vi "HFRR ADV v05.vi"() -> ()   [LabVIEW 2025] (continued)
                        n2289 = property on="Frictional Force ( N )" class="WFChart (strict)"("History Data"=w3345) -> ()  [unwired: 2 in, 2 out]
                        n2290 = property on="Coefficient of Friction" class="WFChart (strict)"("History Data"=w3345) -> ()  [unwired: 2 in, 2 out]
                        n2291 = property on="Frictional Force ( N )" class="WFChart (strict)"("History Data"=w3345) -> ()  [unwired: 2 in, 2 out]
                        n2292 = property on="Electrical Contact Resistance ( % )" class="WFChart (strict)"("History Data"=w3345) -> ()  [unwired: 2 in, 2 out]
                        n2293 = property on="Humidity ( %RH )" class="WFChart (strict)"("History Data"=w3345) -> ()  [unwired: 2 in, 2 out]
                        n2294 = property on="Stroke ( mm )" class="WFChart (strict)"("History Data"=w3346) -> ()  [unwired: 2 in, 2 out]
                        n2295 = property on="Temperature ( Deg C )" class="WFChart (strict)"("History Data"=w3345) -> ()  [unwired: 2 in, 2 out]
                        n2296 = property on="Service Password Log" class="Str"("Visible"=w3347) -> ()  [unwired: 2 in, 2 out]
                        n2297 = property on="Password 3" class="Clust (strict)"("Visible"=w3347) -> ()  [unwired: 2 in, 2 out]
                      }
                    }
                    "TEST FILE NAM,E SAVED" <- TRUE ("TEST FILE NAM,E SAVED")
                  }
                }
              }
            }
          }
        }
        n2298 = case shown="True" w2659 {
          frame False {
            n2299 = local write "tfalg"(0.0 ("tfalg")) -> ()
          }
          frame True {
            n2300 = local read "tfalg"() -> (w2804:dbl)
            n2301 = Equal?(x=w2804, y=0.0) -> (x = y?=w2805:bool)
            n2302 = case shown="True" w2805 {
              frame False {
              }
              frame True {
                n2303 = local read "Total No. of Tests"() -> (w2808:dbl)
                n2304 = local write "tfalg"(1.0 ("tfalg")) -> ()
                n2305 = local write "acq 2"(FALSE ("acq 2")) -> ()
                n2306 = Wait (ms)(milliseconds to wait=u32 200) -> ()  [unwired: 1 out]
                n2307 = Increment(x=w2808) -> (x+1=w2807:dbl)
                n2308 = local write "Total No. of Tests"(w2807) -> ()
              }
            }
          }
        }
        n2309 = local write "Test \nStatus"(w2665) -> ()
        n2310 = local write "Save"(w2665) -> ()
        n2311 = local read "Main Tab"() -> (w2622:T2)
        n2312 = case shown="True" w2646 {
          tunnel: [FALSE ("RUN") TRUE ("RUN")] -> w2645
          tunnel: [_ 1] -> w2638
          frame False {
          }
          frame True {
          }
        }
        n2313 = In Range and Coerce(upper limit=w2653, x=w2626, lower limit=w2652) -> (In Range?=w2644:bool)  [unwired: 1 out]
        n2314 = In Range and Coerce(upper limit=w2650, x=w2625, lower limit=w2651) -> (In Range?=w2642:bool)  [unwired: 1 out]
        n2315 = case shown="True" w2658 {
          frame False {
            n2316 = local read "Rt 3"() -> (w2786:bool)
            n2317 = case shown="True" w2786 {
              frame False {
              }
              frame True {
                n2318 = local write "Rt 3"(FALSE ("Rt 3")) -> ()
                n2319 = local write "Json End Flg"(TRUE ("Upld AR 2")) -> ()
              }
            }
            "Rt" <- TRUE ("Rt")
            "Rt 2" <- FALSE ("Rt")
          }
          frame True {
            n2320 = local read "Rt"() -> (w2793:bool)
            n2321 = local write "Rt 2"(TRUE ("Rt 2")) -> ()
            n2322 = case shown="True" w2793 {
              frame False {
              }
              frame True {
                w2794 = TRUE ("Upld AR 2")
                n2323 = local write "Rt"(FALSE ("Rt")) -> ()
                n2324 = local write "Upld AR"(w2794) -> ()
                n2325 = local write "Json St Flg"(w2794) -> ()
              }
            }
            "Rt 3" <- TRUE ("Rt 3")
          }
        }
        n2326 = case shown="True" w2644 {
          tunnel: [FALSE ("RUN") TRUE ("RUN")] -> w2643
          tunnel: [_ 2] -> w2637
          frame False {
          }
          frame True {
          }
        }
        n2327 = case shown="True" w2642 {
          tunnel: [FALSE ("RUN") TRUE ("RUN")] -> w2641
          tunnel: [_ 3] -> w2636
          frame False {
          }
          frame True {
          }
        }
        n2328 = case shown="\"Acquire\"" w2622 {
          tunnel: w2624 -> [_ w2855]
          frame Default {
            w2854 = 0.0 ("output")
            n2329 = local write "PID-out"(w2854) -> ()
            n2330 = local write "Frequency ( Hz )"(w2854) -> ()
          }
          frame "Acquire" {
            n2331 = stacked-sequence {
              frame #0 {
                n2332 = local read "Auto Start Test"() -> (w2860:bool)
                n2333 = case shown="True" w2860 {
                  tunnel: "RUN" -> [w2880 w2883]
                  tunnel: [w2880 w2882] -> w2861
                  frame False {
                  }
                  frame True {
                    n2334 = local read "Auto Start Temp"() -> (w2881:bool)
                    n2335 = Or(x=w2883, y=w2881) -> (x .or. y?=w2882:bool)
                  }
                }
                n2336 = local read "clk"() -> (w2879:dbl)
                n2337 = local read "Save"() -> (w2875:bool)
                n2338 = Equal?(x=w2879, y=0.0) -> (x = y?=w2876:bool)
                n2339 = And(x=w2876, y=w2875) -> (x .and. y?=w2877:bool)
                n2340 = Not(x="Engage") -> (.not. x?=w2866:bool)
                n2341 = case shown="True" w2861 {
                  tunnel: [0.0 w2900] -> w2858
                  frame False {
                    (unwired) TRUE ("Visible")
                    n2342 = local read "Auto Start Test"() -> (w2887:bool)
                    n2343 = local write "Start Time"(TRUE ("Start Time")) -> ()
                    n2344 = property on="Stroke 2" class="DigNum (strict)"("Visible"=FALSE) -> ()  [unwired: 2 in, 2 out]
                    n2345 = case shown="False" w2887 {
                      frame False {
                        n2346 = property on="Heater Button" class="Bool (strict)"("DisabledEnum"=T13."Enabled" ("Disabled")) -> ()  [unwired: 2 in, 2 out]
                        n2347 = property on="Humidity" class="Bool (strict)"("DisabledEnum"=T13."Enabled" ("Disabled")) -> ()  [unwired: 2 in, 2 out]
                      }
                      frame True {
                      }
                    }
                    n2348 = case shown="False" "TestCompFlg" {
                      frame False {
                        n2349 = local read "StartFlg"() -> (w2895:bool)
                        n2350 = case shown="True" w2895 {
                          frame False {
                          }
                          frame True {
                            n2351 = flat-sequence {
                              frame #0 {
                                n2352 = local read "EVENT LOG"() -> (w2897:string)
                                n2353 = call "Event Log.vi"("Content"="Test was interrupted", "EVENT LOG"=w2897) -> ("EVENT LOG"=w2898:string)  [unwired: 8 in, 1 out]
                                n2354 = local write "EVENT LOG"(w2898) -> ()
                              }
                              frame #1 {
                                w2899 = FALSE ("StartFlg")
                                n2355 = local write "Heater Button"(w2899) -> ()
                                n2356 = local write "StartFlg"(w2899) -> ()
                                n2357 = local write "Humidity"(w2899) -> ()
                              }
                            }
                          }
                        }
                      }
                      frame True {
                      }
                    }
                    n2358 = local write "String 14"("Test will autostart once parameters reach the set value." ("String 14")) -> ()
                  }
                  frame True {
                    (unwired) FALSE ("Visible")
                    n2359 = property on="Stroke 2" class="DigNum (strict)"("Visible"=TRUE) -> ()  [unwired: 2 in, 2 out]
                    n2360 = property on="STOP 2" class="Bool (strict)"("Disabled"=u8 2) -> ()  [unwired: 2 in, 2 out]
                    n2361 = local write "String 14"(" Running....." ("String 14")) -> ()
                    n2362 = property on="Heater Button" class="Bool (strict)"("DisabledEnum"=T13."Disabled and Grayed Out" ("Disabled")) -> ()  [unwired: 2 in, 2 out]
                    n2363 = property on="Humidity" class="Bool (strict)"("DisabledEnum"=T13."Disabled and Grayed Out" ("Disabled")) -> ()  [unwired: 2 in, 2 out]
                    n2364 = case shown="True" "Start Time" {
                      selector: "Start Time" -> [_ w2913]
                      frame False {
                      }
                      frame True {
                        n2365 = Not(x=w2913) -> (.not. x?=w2912:bool)
                        n2366 = local write "Start Time"(w2912) -> ()
                        n2367 = local read "EVENT LOG"() -> (w2914:string)
                        n2368 = call "Event Log.vi"("Content"="Test in progress", "EVENT LOG"=w2914) -> ("EVENT LOG"=w2916:string)  [unwired: 8 in, 1 out]
                        n2369 = local write "EVENT LOG"(w2916) -> ()
                      }
                    }
                    n2370 = local read "Set Hz"() -> (w2910:dbl)
                    n2371 = call <vilib>:"Uniform White Noise Waveform.vi"() -> ("signal out"=w2909:waveform(dbl))  [unwired: 10 in, 1 out]
                    n2372 = Add(x=w2910, y=w2909) -> (x+y=w2908:waveform(dbl))
                    n2373 = Multiply(x=w2908, y=ext 0.1) -> (x*y=w2900:waveform(ext))
                    "StartFlg" <- TRUE ("StartFlg")
                  }
                }
                n2374 = case shown="True" w2877 {
                  frame False {
                  }
                  frame True {
                    n2375 = local write "clk"(10.0 ("clk")) -> ()
                    n2376 = Get Date/Time In Seconds() -> (seconds since 1Jan1904=w2919:timestamp)
                    n2377 = To Double Precision Float(number=w2919) -> (double precision float=w2917:dbl)
                    n2378 = local write "acq timer"(w2917) -> ()
                    n2379 = local write "act save time"(w2917) -> ()
                  }
                }
                n2380 = call "Elapsed Time"("Time Target (s)"="Countdown", "Reset"=w2866) -> ("Elapsed Time (s)"=w2871:dbl, "Time has Elapsed"=w2869:bool)  [unwired: 10 in, 6 out]
                "Countdown 2" <- w2871
                n2381 = Subtract(x=w2871, y=2.0) -> (x-y=w2874:dbl)
                n2382 = Less?(x=w2874, y="Countdown") -> (x < y?=w2872:bool)
                n2383 = And(x=w2872, y=w2869) -> (x .and. y?=w2868:bool)
                n2384 = case shown="True" w2868 {
                  frame False {
                  }
                  frame True {
                    (unwired) dbl[] [] ("History Data")
                    n2385 = local write "Engage"(FALSE ("Engage")) -> ()
                    n2386 = local write "RUN"(TRUE ("RUN")) -> ()
                    n2387 = local read "Humidity ( %RH )"() -> (→"Rh Before":dbl)
                  }
                }
                n2388 = local read "Test \nStatus"() -> (w2864:bool)
                n2389 = Multiply(x=w2858, y=10.0) -> (x*y=w2859:dbl)
                n2390 = Select(t=w2859, s=w2864, f=0.0) -> (s? t:f=w2863:dbl)
                n2391 = local write "Frequency ( Hz )"(w2863) -> ()
              }
              frame #1 {
                w2942 = 1000000.0 ("x")
                # "Elapsed time\ncof\nstroke\nAir temp\nTemp\nHumidity"
                # "acq timer\n\nact save time"
                # "convert to microseconds"
                n2392 = local read "COUNT"() -> (w2925:i32)
                n2393 = local read "Rate"() -> (w2938:dbl)
                n2394 = Divide(x=w2942, y=w2938) -> (x/y=w2943:dbl)
                n2395 = Greater Or Equal?(x=w2925, y=250) -> (x >= y?=w2924:bool)
                n2396 = Get Date/Time In Seconds() -> (seconds since 1Jan1904=w2945:timestamp)
                n2397 = case shown="True" w2924 {
                  frame False {
                    n2398 = local read "COUNT"() -> (w2946:i32)
                    n2399 = Increment(x=w2946) -> (x+1=w2947:i32)
                    n2400 = local write "COUNT"(w2947) -> ()
                  }
                  frame True {
                    n2401 = local write "COUNT"(0 ("COUNT")) -> ()
                  }
                }
                n2402 = local read "Samplingtime 2"() -> (w2923:dbl)
                n2403 = local read "act save time"() -> (w2940:dbl)
                n2404 = Divide(x=w2943, y=w2942) -> (x/y=w2941:dbl)
                n2405 = To Double Precision Float(number=w2945) -> (double precision float=w2934:dbl)
                n2406 = Add(x=w2940, y=w2923) -> (x+y=w2939:dbl)
                n2407 = local read "acq timer"() -> (w2944:dbl)
                n2408 = local read "COUNT"() -> (w2927:i32)
                n2409 = Greater Or Equal?(x=w2934, y=w2939) -> (x >= y?=w2922:bool)
                n2410 = Multiply(x=w2941, y=w2927) -> (x*y=w2933:dbl)
                n2411 = Subtract(x=w2934, y=w2944) -> (x-y=w2936:dbl)
                n2412 = local read "Save"() -> (w2937:bool)
                n2413 = Add(x=w2936, y=w2933) -> (x+y=w2920:dbl)
                "Elapsed time 3" <- w2920
                n2414 = And(x=w2922, y=w2937) -> (x .and. y?=w2935:bool)
                n2415 = Divide(x=w2920, y=60.0) -> (x/y=w2931:dbl)
                n2416 = local read "Test \nStatus"() -> (w2921:bool)
                n2417 = local read "clk"() -> (w2928:dbl)
                n2418 = Equal?(x=w2928, y=10.0) -> (x = y?=w2930:bool)
                n2419 = case shown="True" w2935 {
                  tunnel: w2934 -> [_ w3051]
                  tunnel: [FALSE ("Boolean 2") TRUE ("Boolean 2")] -> _
                  frame False {
                  }
                  frame True {
                    w3005 = ";" ("Substring")
                    # "Pid out/\nFreq response value"
                    n2420 = local write "act save time"(w3051) -> ()
                    n2421 = local read "FILE"() -> (w2999:string)
                    n2422 = call "file check.vi"("file name in"=w2999) -> ("error out"=w3002:errorcluster, "file name out"=w2997:string)  [unwired: 9 in]
                    n2423 = call "FILE PATH CREATION.vi"("error in"=w3002, "FILE NAME :"=w2997) -> ("FILE OUT"=w3000:path)  [unwired: 8 in, 1 out]
                    n2424 = Concatenate Strings(w2997, ".dgf" ("Substring")) -> (w3001:string)
                    n2425 = local read "FF 2"() -> (→"Frictional Force ( N )" →"Frictional Force ( N )":dbl)
                    n2426 = Build Path(base path=w3000, name or relative path=w3001) -> (appended path=w2996:path)
                    n2427 = local read "COF 2"() -> (w3010:dbl)
                    "cof" <- w3010
                    "Coefficient of Friction" <- w3010
                    "COF 4" <- w3010
                    "Coefficient of Friction" <- w3010
                    n2428 = local read "TEMP"() -> (w3013:dbl)
                    "Temp" <- w3013
                    "Temperature ( Deg C )" <- w3013
                    n2429 = local read "Humidity ( %RH )"() -> (w3012:dbl)
                    "Humidity ( %RH )" <- w3012
                    "Humidity ( %RH )" <- w3012
                    n2430 = local read "Frequency ( Hz )"() -> (w3019:dbl)
                    n2431 = local read "Elapsed time"() -> (w3044:dbl)
                    n2432 = local read "AIR TEMP"() -> (w3017:dbl)
                    n2433 = local read "PID-out"() -> (w3022:dbl)
                    n2434 = local write "Temperature ( Deg C )"(w3013) -> ()
                    n2435 = Number To Fractional String(number="measured_stroke", width (-)=i16 9 ("precision (6)"), precision (6)=i16 6) -> (F-format string=w3037:string)  [unwired: 1 in]
                    n2436 = Number To Fractional String(number=w3017, width (-)=i16 9 ("precision (6)"), precision (6)=i16 3) -> (F-format string=w3036:string)  [unwired: 1 in]
                    n2437 = Number To Fractional String(number=w3013, width (-)=i16 9 ("precision (6)"), precision (6)=i16 3) -> (F-format string=w3033:string)  [unwired: 1 in]
                    n2438 = Number To Fractional String(number=w3012, width (-)=i16 9 ("precision (6)"), precision (6)=i16 3) -> (F-format string=w3030:string)  [unwired: 1 in]
                    n2439 = Number To Fractional String(number=0.0, width (-)=i16 9 ("precision (6)"), precision (6)=i16 3) -> (F-format string=w3027:string)  [unwired: 1 in]
                    n2440 = Number To Fractional String(number=w3022, width (-)=i16 9 ("precision (6)"), precision (6)=i16 3) -> (F-format string=w3023:string)  [unwired: 1 in]
                    n2441 = Number To Fractional String(number=w3019, width (-)=i16 9 ("precision (6)"), precision (6)=i16 3) -> (F-format string=w3018:string)  [unwired: 1 in]
                    n2442 = Number To Fractional String(number=w3010, width (-)=i16 9 ("precision (6)"), precision (6)=i16 6) -> (F-format string=w3045:string)  [unwired: 1 in]
                    n2443 = Number To Fractional String(number=w3044, width (-)=i16 14 ("precision (6)"), precision (6)=i16 3) -> (F-format string=w3046:string)  [unwired: 1 in]
                    n2444 = Bundle("y"=1.02, "measured_stroke"="measured_stroke", "y"=0.98) -> (w3011:cluster{"y":dbl, "measured_stroke":dbl, "y":dbl})  [unwired: 1 in]
                    n2445 = Number To Fractional String(number="Ambient Humidity :", width (-)=i16 9 ("precision (6)"), precision (6)=i16 6) -> (F-format string=w3003:string)  [unwired: 1 in]
                    n2446 = local read "RUN"() -> (w3009:bool)
                    n2447 = case shown="True" w3009 {
                      tunnel: w3011 -> [_ w3056]
                      tunnel: "measured_stroke" -> [_ w3055]
                      tunnel: "measured_stroke" -> [_ w3054]
                      tunnel: "measured_stroke" -> [_ w3053]
                      frame False {
                      }
                      frame True {
                        "Stroke ( mm )" <- w3056
                        "Stroke ( mm )" <- w3056
                        "Stroke 4" <- w3055
                        "Stroke 3" <- w3054
                        "Stroke 2" <- w3053
                      }
                    }
                    n2448 = Concatenate Strings(w3046, w3005, w3045, w3005, w3037, w3005, w3036, w3005, w3033, w3005, w3030, w3005, w3027, w3005, w3023, w3005, w3018, w3005, w3003, "\r") -> (w3043:string)
                    n2449 = call <vilib>:"Write Characters To File.vi"("append to file? (new file:F)"=TRUE, "character string"=w3043, "file path (dialog if empty)"=w2996) -> ()  [unwired: 2 in, 1 out]
                    "refresh flag" <- TRUE ("refresh flag")
                  }
                }
                n2450 = case shown="True" w2921 {
                  tunnel: w2931 -> [_ w2957]
                  tunnel: w2936 -> [_ w2967]
                  tunnel: [0.0 w2963] -> _
                  tunnel: w2930 -> [_ w2962]
                  tunnel: [0.0 w2961] -> _
                  tunnel: w2920 -> [_ w2961]
                  tunnel: w2934 -> [w2950 _]
                  frame False {
                    n2451 = local write "acq timer"(w2950) -> ()
                    n2452 = local write "Test Duration Status"(0.0 ("Test Duration Status")) -> ()
                  }
                  frame True {
                    n2453 = local read "Set Hz"() -> (w2964:dbl)
                    n2454 = local write "Elapsed time"(w2957) -> ()
                    n2455 = local read "test time"() -> (w2956:dbl)
                    n2456 = Multiply(x=w2967, y=w2964) -> (x*y=w2966:dbl)
                    n2457 = case shown="False" w2962 {
                      tunnel: w2966 -> [w2968 _]
                      tunnel: [w2968 1.0] -> w2963
                      frame False {
                        n2458 = local write "Cycles elapsed"(w2968) -> ()
                      }
                      frame True {
                      }
                    }
                    n2459 = Greater?(x=w2957, y=w2956) -> (0:w2965:bool)
                    n2460 = Subtract(x=w2956, y=w2957) -> (x-y=w2955:dbl)
                    "time" <- w2955
                    n2461 = Multiply(x=w2955, y=60.0) -> (x*y=w2954:dbl)
                    n2462 = local write "Time Remaining"(w2954) -> ()
                    n2463 = local write "Remaining Time"(w2954) -> ()
                    n2464 = case shown="True" w2965 {
                      frame False {
                      }
                      frame True {
                        n2465 = stacked-sequence {
                          frame #0 {
                            w2971 = T13."Enabled" ("Disabled")
                            w2970 = FALSE ("TEST FILE NAM,E SAVED")
                            w2974 = "" ("FILE")
                            w2975 = TRUE ("Visible")
                            n2466 = local write "Humidity"(FALSE ("Humidity")) -> ()
                            n2467 = local write "RUN"(FALSE ("OK Button 2")) -> ()
                            n2468 = local write "Heater Button"(FALSE ("Heater Button")) -> ()
                            n2469 = local write "Auto Start Test"(FALSE ("Auto Start Test")) -> ()
                            n2470 = local write "TestCompFlg"(TRUE ("StpFlg")) -> ()
                            n2471 = local read "Humidity ( %RH )"() -> (→"Rh After":dbl)
                            n2472 = property on="STOP 2" class="Bool (strict)"("Disabled"=u8 0) -> ()  [unwired: 2 in, 2 out]
                            n2473 = local read "EVENT LOG"() -> (w2980:string)
                            n2474 = call "Event Log.vi"("Content"="Test Completed", "EVENT LOG"=w2980) -> ("EVENT LOG"=w2979:string)  [unwired: 8 in, 1 out]
                            n2475 = property on="RUN" class="Bool (strict)"("Visible"=w2975) -> ()  [unwired: 2 in, 2 out]
                            n2476 = property on="Auto Start Test" class="Bool (strict)"("Visible"=w2975) -> ()  [unwired: 2 in, 2 out]
                            n2477 = local write "Batch Ref Num :"(w2974) -> ()
                            n2478 = local write "FILE"(w2974) -> ()
                            n2479 = local write "EVENT LOG"(w2979) -> ()
                            n2480 = local write "TEST FILE NAM,E SAVED"(w2970) -> ()
                            n2481 = local write "Fuel Discription :"(w2974) -> ()
                            n2482 = local write "START TEMP"(w2970) -> ()
                            n2483 = local write "Remarks :"(w2974) -> ()
                            n2484 = local write "Main Dashboard Buttons"(T1."Imaging" ("Main Dashboard Buttons")) -> ()
                            n2485 = local write "Main Tab"(T2."Adv Scar" ("Main Tab")) -> ()
                            n2486 = property on="FRICVALZ 2" class="Bool (strict)"("DisabledEnum"=w2971) -> ()  [unwired: 2 in, 2 out]
                            n2487 = property on="FRICVALZ 3" class="Bool (strict)"("DisabledEnum"=w2971) -> ()  [unwired: 2 in, 2 out]
                            n2488 = property on="FRICVALZ 4" class="Bool (strict)"("DisabledEnum"=w2971) -> ()  [unwired: 2 in, 2 out]
                          }
                          frame #1 {
                            n2489 = Wait (ms)(milliseconds to wait=u32 1500) -> ()  [unwired: 1 out]
                          }
                          frame #2 {
                            n2490 = local write "Command"("VC;0") -> ()
                          }
                          frame #3 {
                            n2491 = Wait (ms)(milliseconds to wait=u32 1500) -> ()  [unwired: 1 out]
                          }
                          frame #4 {
                            n2492 = local write "Command"("ST;0") -> ()
                          }
                          frame #5 {
                            n2493 = Wait (ms)(milliseconds to wait=u32 1500) -> ()  [unwired: 1 out]
                          }
                          frame #6 {
                            n2494 = local write "Command"("HE;0" ("Command")) -> ()
                          }
                          frame #7 {
                            n2495 = Wait (ms)(milliseconds to wait=u32 1500) -> ()  [unwired: 1 out]
                          }
                        }
                      }
                    }
                    n2496 = Divide(x=w2957, y=w2956) -> (x/y=w2960:dbl)
                    n2497 = Multiply(x=w2960, y=100.0) -> (x*y=w2958:dbl)
                    n2498 = local write "Test Duration Status"(w2958) -> ()
                  }
                }
              }
              frame #2 {
                n2499 = case shown="True" "Heater Button" {
                  tunnel: [0.0 ("output") w3066] -> w3057
                  frame False {
                    w3060 = TRUE ("tmpchk")
                    n2500 = local read "TEMP"() -> (w3061:dbl)
                    n2501 = local write "Temp ini"(w3061) -> ()
                    n2502 = local write "Reset 4"(w3060) -> ()
                    n2503 = local write "tmpchk"(w3060) -> ()
                    n2504 = local write "reinit"(TRUE ("reinit")) -> ()
                    n2505 = local write "manual temp log"(TRUE ("manual temp log")) -> ()
                  }
                  frame True {
                    n2506 = local read "Auto Start Test"() -> (w3065:bool)
                    n2507 = case shown="True" FALSE {
                      tunnel: [_ w3081] -> w3066
                      frame False {
                      }
                      frame True {
                        # "Logic to turn off\nthe heater when \ntemp is not rising.\nTime - 60 sec\nDelta t- 5°c"
                        n2508 = local read "Temp ini"() -> (w3070:dbl)
                        n2509 = Less?(x=w3070, y=53.0) -> (x < y?=w3068:bool)
                        n2510 = And(x="tmpchk", y=w3068) -> (x .and. y?=w3071:bool)
                        n2511 = case shown="True" w3071 {
                          frame False {
                          }
                          frame True {
                            n2512 = call "Elapsed Time8"("Time Target (s)"=300.0, "Reset"="Reset 4") -> ("Time has Elapsed"=w3084:bool)  [unwired: 10 in, 7 out]
                            n2513 = flat-sequence {
                              tunnel: w3084 -> [_]
                              frame #0 {
                                n2514 = local write "Reset 4"(FALSE ("Reset 4")) -> ()
                              }
                            }
                            n2515 = case shown="True" w3084 {
                              frame False {
                              }
                              frame True {
                                n2516 = local read "Temp ini"() -> (w3091:dbl)
                                n2517 = Add(x=w3091, y=5.0) -> (x+y=w3089:dbl)
                                n2518 = local read "TEMP"() -> (w3092:dbl)
                                n2519 = Greater?(x=w3092, y=w3089) -> (0:w3090:bool)
                                n2520 = case shown="False" w3090 {
                                frame False {
                                n2521 = local write "Heater Button"(FALSE ("Heater Button")) -> ()
                                }
                                frame True {
                                n2522 = local write "tmpchk"(FALSE ("tmpchk")) -> ()
                                }
                                }
                              }
                            }
                          }
                        }
                        n2523 = local read "Set Temp"() -> (w3079:dbl)
                        n2524 = local read "TEMP"() -> (w3073:dbl)
                        n2525 = call-poly <vilib>:"PID.vi"("reinitialize? (F)"="reinit", "dt (s)"=-1.0, "process variable"=w3073, "setpoint"=w3079) -> ("output"=w3076:dbl)  [unwired: 6 in, 1 out]
                        n2526 = Subtract(x=w3079, y=w3073) -> (x-y=w3080:dbl)
                        n2527 = Add(x=w3079, y=0.5) -> (x+y=w3077:dbl)
                        n2528 = Greater Or Equal?(x=w3073, y=w3077) -> ()  [unwired: 1 out]
                        n2529 = Select(t=0.0, s=FALSE, f=w3076) -> (s? t:f=w3075:dbl)
                        "PID output" <- w3075
                        n2530 = flat-sequence {
                          tunnel: w3075 -> [w3095]
                          tunnel: [w3095] -> w3081
                          frame #0 {
                            n2531 = local write "reinit"(FALSE ("reinit")) -> ()
                          }
                        }
                        n2532 = Bundle(w3080, "output"=w3075, "TEMP"=w3073) -> ()  [unwired: 1 in, 1 out]
                      }
                    }
                    n2533 = case shown="False" w3065 {
                      frame False {
                        n2534 = local read "Set Temp"() -> (w3103:dbl)
                        n2535 = local read "TEMP"() -> (w3102:dbl)
                        n2536 = Subtract(x=w3103, y=w3102) -> (x-y=w3101:dbl)
                        n2537 = Absolute Value(x=w3101) -> (abs(x)=w3100:dbl)
                        n2538 = Less?(x=w3100, y=0.5) -> (x < y?=w3098:bool)
                        n2539 = case shown="True" w3098 {
                          tunnel: "manual temp log" -> [_ w3104]
                          frame False {
                          }
                          frame True {
                            n2540 = case shown="True" w3104 {
                              selector: w3104 -> [_ w3105]
                              frame False {
                              }
                              frame True {
                                # "#Event log"
                                n2541 = Not(x=w3105) -> (.not. x?=w3106:bool)
                                n2542 = local write "manual temp log"(w3106) -> ()
                                n2543 = local read "EVENT LOG"() -> (w3109:string)
                                n2544 = call "Event Log.vi"("Content"="Target Temperature reached", "EVENT LOG"=w3109) -> ("EVENT LOG"=w3108:string)  [unwired: 8 in, 1 out]
                                n2545 = local write "EVENT LOG"(w3108) -> ()
                              }
                            }
                          }
                        }
                      }
                      frame True {
                        n2546 = local write "manual temp log"(TRUE ("manual temp log")) -> ()
                      }
                    }
                  }
                }
                "PID-out" <- w3057
              }
              frame #3 {
                n2547 = local read "TEMP"() -> (w3111:dbl)
                n2548 = Greater Or Equal?(x=w3111, y="Set Temp 2") -> (x >= y?=w3116:bool)
                n2549 = case shown="True" w3116 {
                  tunnel: [FALSE TRUE] -> w3114
                  frame False {
                  }
                  frame True {
                  }
                }
                "Status 13" <- w3114
                n2550 = And(x=w3114, y="trip1 8") -> (x .and. y?=w3113:bool)
                n2551 = case shown="True" w3113 {
                  frame False {
                    n2552 = local write "Heater Trip Temp"(TRUE ("Heater Trip Temp")) -> ()
                  }
                  frame True {
                    w3119 = FALSE ("OK Button 2")
                    n2553 = case shown="True" "Heater Trip Temp" {
                      selector: "Heater Trip Temp" -> [_ w3121]
                      frame False {
                      }
                      frame True {
                        n2554 = Not(x=w3121) -> (.not. x?=w3120:bool)
                        n2555 = local read "EVENT LOG"() -> (w3124:string)
                        n2556 = local write "Heater Trip Temp"(w3120) -> ()
                        n2557 = call "Event Log.vi"("Content"="Heater Trip", "EVENT LOG"=w3124) -> ("EVENT LOG"=w3123:string)  [unwired: 8 in, 1 out]
                        n2558 = local write "EVENT LOG"(w3123) -> ()
                      }
                    }
                    n2559 = local write "RUN"(w3119) -> ()
                    n2560 = property on="Auto Start Test" class="Bool (strict)"("Value"=w3119) -> ()  [unwired: 2 in, 2 out]
                    n2561 = local write "Heater Button"(w3119) -> ()
                  }
                }
              }
            }
            n2562 = case shown="False" w2855 {
              frame False {
                n2563 = disable-structure shown="Enabled" {
                  frame Disabled {
                    n2564 = stacked-sequence {
                      frame #0 {
                        n2565 = local write "RUN"(FALSE ("OK Button 2")) -> ()
                      }
                      frame #1 {
                      }
                    }
                  }
                  frame Enabled {
                  }
                }
              }
              frame True {
              }
            }
          }
        }
        n2566 = local read "airtempflg"() -> (w2647:bool)
        n2567 = Or(x=w2647, y=w2645) -> (x .or. y?=w2648:bool)
        n2568 = Insert Into Array(array=string[] ["Air Temperature has reached set value,", "Humidity has reached set value,", "Sample Temperaturehas reached set value,", ""], index=0, new element="") -> (w2633:string[])
        n2569 = Build Array(w2638, w2637, w2636) -> (w2634:i32[])
        n2570 = disable-structure shown="Disabled" {
          disable-tunnel: w2648 -> [w2725 _]
          disable-tunnel: w2643 -> [w2724 _]
          disable-tunnel: w2641 -> [w2723 _]
          frame Disabled {
            n2571 = Compound Arithmetic op=AND(w2725, w2724, w2723) -> ()  [unwired: 1 out]
            n2572 = case shown="True" {
              selector: _ -> [_ _]
              frame False {
              }
              frame True {
                w2726 = FALSE ("autostrtflg")
                n2573 = local write "RUN"(TRUE ("RUN")) -> ()
                n2574 = local write "autostrtflg"(w2726) -> ()
                n2575 = local write "autostart"(w2726) -> ()
                n2576 = local write "String 14"(" Running....." ("String 14")) -> ()
              }
            }
          }
          frame Enabled {
          }
        }
        n2577 = for {
          tunnel: w2634 -> [w2776] mode=indexing
          tunnel: w2633 -> [w2775]
          shift-right: [w2772] -> w2632
          shift-left: "" -> [w2774]
          n2578 = Index Array(array=w2775, index=w2776) -> (element=w2773:string)
          n2579 = Concatenate Strings(w2773, w2774) -> (w2772:string)
        }
        n2580 = local write "autostart 2"(w2632) -> ()
        n2581 = local read "Reset Graph"() -> (w2621:bool)
        n2582 = case shown="True" w2621 {
          selector: w2621 -> [_ w2675]
          frame False {
          }
          frame True {
            w2689 = 0.0 ("X Scale.Range:Maximum")
            n2583 = Not(x=w2675) -> (.not. x?=w2674:bool)
            n2584 = local write "Reset Graph"(w2674) -> ()
            n2585 = property on="Electrical Contact Resistance ( % )" class="WFChart (strict)"("XScale.Maximum"=600.0 ("X Scale.Range:Maximum"), "XScale.Minimum"=0.0 ("X Scale.Range:Minimum"), "YScale.Maximum"=100.0 ("Y Scale.Range:Maximum"), "YScale.Minimum"=0.0 ("Y Scale.Range:Minimum")) -> ()  [unwired: 2 in, 2 out]
            n2586 = property on="Frictional Force ( N )" class="WFChart (strict)"("XScale.Maximum"=600.0 ("X Scale.Range:Maximum"), "XScale.Minimum"=0.0 ("X Scale.Range:Minimum"), "YScale.Maximum"=100.0 ("Y Scale.Range:Maximum"), "YScale.Minimum"=0.0 ("Y Scale.Range:Minimum")) -> ()  [unwired: 2 in, 2 out]
            n2587 = property on="Temperature ( Deg C )" class="WFChart (strict)"("XScale.Maximum"=600.0 ("X Scale.Range:Maximum"), "XScale.Minimum"=0.0 ("X Scale.Range:Minimum"), "YScale.Maximum"=100.0 ("Y Scale.Range:Maximum"), "YScale.Minimum"=0.0 ("Y Scale.Range:Minimum")) -> ()  [unwired: 2 in, 2 out]
            n2588 = property on="Humidity ( %RH )" class="WFChart (strict)"("XScale.Maximum"=600.0 ("X Scale.Range:Maximum"), "XScale.Minimum"=0.0 ("X Scale.Range:Minimum"), "YScale.Maximum"=100.0 ("Y Scale.Range:Maximum"), "YScale.Minimum"=0.0 ("Y Scale.Range:Minimum")) -> ()  [unwired: 2 in, 2 out]
            n2589 = property on="Stroke ( mm )" class="WFChart (strict)"("XScale.Maximum"=600.0 ("X Scale.Range:Maximum"), "XScale.Minimum"=0.0 ("X Scale.Range:Minimum"), "YScale.Maximum"=100.0 ("Y Scale.Range:Maximum"), "YScale.Minimum"=0.0 ("Y Scale.Range:Minimum")) -> ()  [unwired: 2 in, 2 out]
            n2590 = property on="Coefficient of Friction" class="WFChart (strict)"("XScale.Maximum"=600.0 ("X Scale.Range:Maximum"), "XScale.Minimum"=0.0 ("X Scale.Range:Minimum"), "YScale.Maximum"=100.0 ("Y Scale.Range:Maximum"), "YScale.Minimum"=0.0 ("Y Scale.Range:Minimum")) -> ()  [unwired: 2 in, 2 out]
            n2591 = property on="Electrical Contact Resistance ( % )" class="WFChart (strict)"("XScale.Minimum"=0.0 ("X Scale.Range:Minimum"), "XScale.Maximum"=600.0 ("X Scale.Range:Maximum"), "YScale.Minimum"=0.0 ("Y Scale.Range:Minimum"), "YScale.Maximum"=100.0 ("Y Scale.Range:Maximum")) -> ()  [unwired: 2 in, 2 out]
            n2592 = property on="Temperature ( Deg C )" class="WFChart (strict)"("XScale.Minimum"=0.0 ("X Scale.Range:Minimum"), "XScale.Maximum"=600.0 ("X Scale.Range:Maximum"), "YScale.Minimum"=0.0 ("Y Scale.Range:Minimum"), "YScale.Maximum"=100.0 ("Y Scale.Range:Maximum")) -> ()  [unwired: 2 in, 2 out]
            n2593 = property on="Coefficient of Friction" class="WFChart (strict)"("XScale.Minimum"=0.0 ("X Scale.Range:Minimum"), "XScale.Maximum"=600.0 ("X Scale.Range:Maximum"), "YScale.Maximum"=1.0 ("X Scale.Range:Minimum"), "YScale.Minimum"=0.0 ("X Scale.Range:Minimum")) -> ()  [unwired: 2 in, 2 out]
            n2594 = property on="Frictional Force ( N )" class="WFChart (strict)"("XScale.Maximum"=600.0 ("X Scale.Range:Maximum"), "XScale.Minimum"=w2689, "YScale.Maximum"=10.0 ("Y Scale.Range:Maximum"), "YScale.Minimum"=w2689) -> ()  [unwired: 2 in, 2 out]
            n2595 = property on="Stroke ( mm )" class="WFChart (strict)"("XScale.Maximum"=600.0 ("X Scale.Range:Maximum"), "XScale.Minimum"=0.0 ("X Scale.Range:Minimum"), "YScale.Maximum"=100.0 ("Y Scale.Range:Maximum"), "YScale.Minimum"=0.0 ("Y Scale.Range:Minimum")) -> ()  [unwired: 2 in, 2 out]
            n2596 = property on="Humidity ( %RH )" class="WFChart (strict)"("XScale.Maximum"=600.0 ("X Scale.Range:Maximum"), "XScale.Minimum"=0.0 ("X Scale.Range:Minimum"), "YScale.Maximum"=100.0 ("Y Scale.Range:Maximum"), "YScale.Minimum"=0.0 ("Y Scale.Range:Minimum")) -> ()  [unwired: 2 in, 2 out]
          }
        }
      }
      frame "Compare Files" {
        # "Elapsed time\ncof\nstroke\nAir temp\nTemp\nHumidity"
        n2597 = case shown="True" "RSTV1 2" {
          frame False {
          }
          frame True {
            n2598 = property on="Humidity ( %RH )" class="XYGraph (strict)"("Y Scale.Display Format:Precision"=u8 0 ("Y Scale.Format & Precision:Precision")) -> ()  [unwired: 2 in, 2 out]
            n2599 = property on="Humidity ( %RH )" class="XYGraph (strict)"("X Scale.Range:Minimum"=0.0, "X Scale.Range:Maximum"=75.0, "Y Scale.Range:Minimum"=48.0, "Y Scale.Range:Maximum"=58.0) -> ()  [unwired: 2 in, 2 out]
          }
        }
        n2600 = case shown="True" "RST CP 2" {
          frame False {
          }
          frame True {
            n2601 = property on="XY Graph 13" class="XYGraph (strict)"("Y Scale.Display Format:Precision"=u8 0 ("Y Scale.Format & Precision:Precision")) -> ()  [unwired: 2 in, 2 out]
            n2602 = property on="XY Graph 13" class="XYGraph (strict)"("X Scale.Range:Minimum"=0.0, "X Scale.Range:Maximum"=75.0, "Y Scale.Range:Minimum"=0.0, "Y Scale.Range:Maximum"=100.0) -> ()  [unwired: 2 in, 2 out]
          }
        }
        n2603 = case shown="True" "RST CP" {
          frame False {
          }
          frame True {
            n2604 = property on="Sample Temperature ( °C )" class="XYGraph (strict)"("Y Scale.Display Format:Precision"=u8 2 ("Y Scale.Format & Precision:Precision")) -> ()  [unwired: 2 in, 2 out]
            n2605 = property on="Sample Temperature ( °C )" class="XYGraph (strict)"("X Scale.Range:Minimum"=0.0, "X Scale.Range:Maximum"=75.0, "Y Scale.Range:Minimum"=58.0, "Y Scale.Range:Maximum"=62.0) -> ()  [unwired: 2 in, 2 out]
          }
        }
        n2606 = case shown="True" "RSTV1 3" {
          frame False {
          }
          frame True {
            n2607 = property on="Air Temperature  ( °C )" class="XYGraph (strict)"("Y Scale.Display Format:Precision"=u8 2 ("Y Scale.Format & Precision:Precision")) -> ()  [unwired: 2 in, 2 out]
            n2608 = property on="Air Temperature  ( °C )" class="XYGraph (strict)"("X Scale.Range:Minimum"=0.0 ("Y Scale.Range:Minimum"), "X Scale.Range:Maximum"=75.0 ("Y Scale.Range:Maximum"), "Y Scale.Range:Minimum"=20.0 ("X Scale.Range:Minimum"), "Y Scale.Range:Maximum"=26.0 ("X Scale.Range:Maximum")) -> ()  [unwired: 2 in, 2 out]
          }
        }
        n2609 = case shown="True" "RSTV1 4" {
          frame False {
          }
          frame True {
            n2610 = property on="Stroke ( mm )" class="XYGraph (strict)"("Y Scale.Display Format:Precision"=u8 2 ("Y Scale.Format & Precision:Precision")) -> ()  [unwired: 2 in, 2 out]
            n2611 = property on="Stroke ( mm )" class="XYGraph (strict)"("X Scale.Range:Minimum"=0.0 ("Y Scale.Range:Maximum"), "X Scale.Range:Maximum"=75.0 ("X Scale.Range:Minimum"), "Y Scale.Range:Minimum"=0.98, "Y Scale.Range:Maximum"=1.02) -> ()  [unwired: 2 in, 2 out]
          }
        }
        n2612 = case shown="True" "rstv2" {
          frame False {
          }
          frame True {
            n2613 = property on="Coefficient Of Friction" class="XYGraph (strict)"("Y Scale.Display Format:Precision"=u8 3 ("Y Scale.Format & Precision:Precision")) -> ()  [unwired: 2 in, 2 out]
            n2614 = property on="Coefficient Of Friction" class="XYGraph (strict)"("X Scale.Range:Minimum"=0.0 ("Y Scale.Range:Maximum"), "X Scale.Range:Maximum"=75.0, "Y Scale.Range:Minimum"=0.0, "Y Scale.Range:Maximum"=1.0 ("X Scale.Range:Minimum")) -> ()  [unwired: 2 in, 2 out]
          }
        }
        n2615 = case shown="True" "RST CP 3" {
          frame False {
          }
          frame True {
            n2616 = property on="Air Temp ( °C ) vs Humidity ( % RH )" class="XYGraph (strict)"("X Scale.Range:Minimum"=18.0, "X Scale.Range:Maximum"=28.0 ("X Scale.Range:Minimum"), "Y Scale.Range:Minimum"=30.0 ("X Scale.Range:Minimum"), "Y Scale.Range:Maximum"=70.0 ("X Scale.Range:Minimum")) -> ()  [unwired: 2 in, 2 out]
          }
        }
        n2617 = case shown="True" "OPEN 1" {
          frame False {
          }
          frame True {
            (unwired) 0  # existing file
            w3400 = "Choose a datalog file to open"  # prompt
            n2618 = local write "OPEN 1"(FALSE ("OPEN 1")) -> ()
            n2619 = String To Path(string="C:\\LAB-IQ\\Data\\") -> (path=w3385:path)
            n2620 = File Dialog(6:"*.dgf" ("pattern"), 7:w3400, 11:w3385) -> (0:w3383:errorcluster, 3:w3391:path)  [unwired: 4 in, 2 out]
            n2621 = Unbundle(w3383) -> ()  [unwired: 3 out]
            n2622 = Strip Path(path=w3391) -> (name=w3390:string)  [unwired: 1 out]
            n2623 = Path To String(path=w3391) -> (string=w3386:string)
            "string1" <- w3386
            n2624 = Match Pattern(string=w3390, regular expression=".dgf") -> (before substring=→"String Control":string)  [unwired: 1 in, 3 out]
            n2625 = Match Pattern(string=w3386, regular expression=".dgf" ("substring (\"\")")) -> (before substring=w3396:string)  [unwired: 1 in, 3 out]
            n2626 = Concatenate Strings(w3396, ".duf" ("Substring")) -> (w3392:string)
            n2627 = String To Path(string=w3392) -> (path=w3397:path)
            n2628 = call <vilib>:"Read Characters From File.vi"("file path (dialog if empty)"=w3397, "start of read offset (chars.:0)"=60 ("start of read offset (chars.: 0)")) -> ("character string"=→"String Control 2":string)  [unwired: 4 in, 3 out]
          }
        }
        n2629 = case shown="True" "OPEN 2" {
          frame False {
          }
          frame True {
            (unwired) 0  # existing file
            w3418 = "Choose a datalog file to open"  # prompt
            n2630 = local write "OPEN 2"(FALSE ("OPEN 1")) -> ()
            n2631 = String To Path(string="C:\\LAB-IQ\\Data\\") -> (path=w3403:path)
            n2632 = File Dialog(6:"*.dgf" ("pattern"), 7:w3418, 11:w3403) -> (0:w3401:errorcluster, 3:w3409:path)  [unwired: 4 in, 2 out]
            n2633 = Unbundle(w3401) -> ()  [unwired: 3 out]
            n2634 = Strip Path(path=w3409) -> (name=w3407:string)  [unwired: 1 out]
            n2635 = Path To String(path=w3409) -> (string=w3404:string)
            "string1 2" <- w3404
            n2636 = Match Pattern(string=w3407, regular expression=".dgf") -> (before substring=→"String Control 3":string)  [unwired: 1 in, 3 out]
            n2637 = Match Pattern(string=w3404, regular expression=".dgf" ("substring (\"\")")) -> (before substring=w3415:string)  [unwired: 1 in, 3 out]
            n2638 = Concatenate Strings(w3415, ".duf" ("Substring")) -> (w3412:string)
            n2639 = String To Path(string=w3412) -> (path=w3410:path)
            n2640 = call <vilib>:"Read Characters From File.vi"("file path (dialog if empty)"=w3410, "start of read offset (chars.:0)"=60 ("start of read offset (chars.: 0)")) -> ("character string"=→"String Control 4":string)  [unwired: 4 in, 3 out]
          }
        }
        n2641 = case shown="True" "OPEN 3" {
          frame False {
          }
          frame True {
            (unwired) 0  # existing file
            w3436 = "Choose a datalog file to open"  # prompt
            n2642 = local write "OPEN 3"(FALSE ("OPEN 1")) -> ()
            n2643 = String To Path(string="C:\\LAB-IQ\\Data\\") -> (path=w3421:path)
            n2644 = File Dialog(6:"*.dgf" ("pattern"), 7:w3436, 11:w3421) -> (0:w3419:errorcluster, 3:w3427:path)  [unwired: 4 in, 2 out]
            n2645 = Unbundle(w3419) -> ()  [unwired: 3 out]
            n2646 = Strip Path(path=w3427) -> (name=w3425:string)  [unwired: 1 out]
            n2647 = Path To String(path=w3427) -> (string=w3422:string)
            "string1 3" <- w3422
            n2648 = Match Pattern(string=w3425, regular expression=".dgf") -> (before substring=→"String Control 5":string)  [unwired: 1 in, 3 out]
            n2649 = Match Pattern(string=w3422, regular expression=".dgf" ("substring (\"\")")) -> (before substring=w3432:string)  [unwired: 1 in, 3 out]
            n2650 = Concatenate Strings(w3432, ".duf" ("Substring")) -> (w3429:string)
            n2651 = String To Path(string=w3429) -> (path=w3433:path)
            n2652 = call <vilib>:"Read Characters From File.vi"("file path (dialog if empty)"=w3433, "start of read offset (chars.:0)"=60 ("start of read offset (chars.: 0)")) -> ("character string"=→"String Control 6":string)  [unwired: 4 in, 3 out]
          }
        }
        n2653 = case shown="True" "OPEN 4" {
          frame False {
          }
          frame True {
            (unwired) 0  # existing file
            w3454 = "Choose a datalog file to open"  # prompt
            n2654 = local write "OPEN 4"(FALSE ("OPEN 1")) -> ()
            n2655 = String To Path(string="C:\\LAB-IQ\\Data\\") -> (path=w3439:path)
            n2656 = File Dialog(6:"*.dgf" ("pattern"), 7:w3454, 11:w3439) -> (0:w3437:errorcluster, 3:w3445:path)  [unwired: 4 in, 2 out]
            n2657 = Unbundle(w3437) -> ()  [unwired: 3 out]
            n2658 = Strip Path(path=w3445) -> (name=w3443:string)  [unwired: 1 out]
            n2659 = Path To String(path=w3445) -> (string=w3440:string)
            "string1 4" <- w3440
            n2660 = Match Pattern(string=w3443, regular expression=".dgf") -> (before substring=→"String Control 7":string)  [unwired: 1 in, 3 out]
            n2661 = Match Pattern(string=w3440, regular expression=".dgf" ("substring (\"\")")) -> (before substring=w3450:string)  [unwired: 1 in, 3 out]
            n2662 = Concatenate Strings(w3450, ".duf" ("Substring")) -> (w3447:string)
            n2663 = String To Path(string=w3447) -> (path=w3451:path)
            n2664 = call <vilib>:"Read Characters From File.vi"("file path (dialog if empty)"=w3451, "start of read offset (chars.:0)"=60 ("start of read offset (chars.: 0)")) -> ("character string"=→"String Control 8":string)  [unwired: 4 in, 3 out]
          }
        }
      }
      frame "About" {
        # "Elapsed time\ncof\nstroke\nmean pos\nTemp\nHumidity"
        n2665 = disable-structure shown="Disabled" {
          frame Disabled {
            n2666 = case shown="True" "Export" {
              frame False {
              }
              frame True {
                w3476 = "                                      " ("string")
                w3478 = "\r"
                (unwired) i16 6 ("width (-)")
                w3555 = "\r"
                w3487 = "\r"
                n2667 = local write "Export"(FALSE ("Export")) -> ()
                n2668 = local read "String 29"() -> (w3524:string)
                n2669 = local read "String 34"() -> (w3512:string)
                n2670 = local read "String 35"() -> (w3507:string)
                n2671 = local read "String 37"() -> (w3503:string)
                n2672 = local read "String 36"() -> (w3500:string)
                n2673 = local read "String 38"() -> (w3497:string)
                n2674 = local read "String 39"() -> (w3494:string)
                n2675 = Match Pattern(string=w3524, regular expression=".dwm") -> (before substring=w3520:string)  [unwired: 1 in, 3 out]
                "before substring" <- w3520
                n2676 = local read "S 38"() -> (w3515:string)
                n2677 = local read "S 39"() -> (w3508:string)
                n2678 = local read "Temperature before test 2"() -> (w3544:dbl)
                n2679 = local read "Temperature after test 2"() -> (w3549:dbl)
                n2680 = local read "Humidity before test 2"() -> (w3530:dbl)
                n2681 = local read "Humidity after test 2"() -> (w3545:dbl)
                n2682 = local read "MWSD 2"() -> (w3541:dbl)
                n2683 = local read "WS1.4 2"() -> (w3557:dbl)
                n2684 = local read "HCF 2"() -> (w3553:dbl)
                n2685 = local read "AVP 2"() -> (w3542:dbl)
                n2686 = Concatenate Strings("1," ("string"), w3515) -> (w3514:string)
                n2687 = Concatenate Strings("2," ("string"), w3512) -> (w3511:string)
                n2688 = Concatenate Strings("3," ("string"), w3508) -> (w3510:string)
                n2689 = Concatenate Strings("4," ("string"), w3507) -> (w3506:string)
                n2690 = Concatenate Strings("5," ("string"), w3503) -> (w3504:string)
                n2691 = Concatenate Strings("6," ("string"), w3500) -> (w3501:string)
                n2692 = Concatenate Strings("7," ("string"), w3497) -> (w3498:string)
                n2693 = Concatenate Strings("8," ("string"), w3494) -> (w3495:string)
                n2694 = local read "Sample ID"() -> (w3562:string)
                n2695 = case shown="\"xlx\"" "Select File Type" {
                  tunnel: w3520 -> [w3565 w3567 w3569]
                  tunnel: [w3563 w3568 w3570] -> w3519
                  frame "xlx" {
                    n2696 = Concatenate Strings(w3565, ".xls" ("string")) -> (w3563:string)
                  }
                  frame "csv" {
                    n2697 = Concatenate Strings(w3567, ".csv" ("string")) -> (w3568:string)
                  }
                  frame "txt" {
                    n2698 = Concatenate Strings(w3569, ".txt" ("string")) -> (w3570:string)
                  }
                }
                n2699 = local read "Test Date"() -> (w3561:string)
                n2700 = local read "String 45"() -> (w3475:string)
                n2701 = local read "String 31"() -> (w3560:string)
                n2702 = local read "String 32"() -> (w3559:string)
                n2703 = local read "TITTLE"() -> (w3483:string)
                n2704 = Number To Fractional String(number=w3530, width (-)=i16 6, precision (6)=i16 2) -> (F-format string=w3529:string)  [unwired: 1 in]
                n2705 = Number To Fractional String(number=w3544, width (-)=i16 6, precision (6)=i16 2) -> (F-format string=w3550:string)  [unwired: 1 in]
                n2706 = Number To Fractional String(number=w3545, width (-)=i16 6, precision (6)=i16 2) -> (F-format string=w3543:string)  [unwired: 1 in]
                n2707 = Number To Fractional String(number=w3549, width (-)=i16 6, precision (6)=i16 2) -> (F-format string=w3548:string)  [unwired: 1 in]
                n2708 = Number To Fractional String(number=w3541, width (-)=i16 6, precision (6)=i16 2) -> (F-format string=w3539:string)  [unwired: 1 in]
                n2709 = Number To Fractional String(number=w3542, width (-)=i16 6, precision (6)=i16 2) -> (F-format string=w3540:string)  [unwired: 1 in]
                n2710 = Number To Fractional String(number=w3553, width (-)=i16 6, precision (6)=i16 2) -> (F-format string=w3554:string)  [unwired: 1 in]
                n2711 = Number To Fractional String(number=w3557, precision (6)=i16 2) -> (F-format string=w3558:string)  [unwired: 2 in]
                n2712 = local read "s.NO"() -> (w3477:string)
                n2713 = Concatenate Strings("=" ("string"), w3483) -> (w3482:string)
                n2714 = Concatenate Strings("S.No," ("string"), "                                       Parameters" ("string")) -> (w3488:string)
                n2715 = Concatenate Strings(w3555, w3514, w3529, w3555, w3511, w3550, w3555, w3510, w3543, w3555, w3506, w3548, w3555, w3504, w3539, w3555, w3501, w3540, w3555, w3498, w3554, w3555, w3495, w3558) -> (w3517:string)
                n2716 = Concatenate Strings(w3487, "," ("string"), w3475, w3477, w3476, w3559, w3562, w3476, w3560, w3561, w3487) -> (w3485:string)
                n2717 = local read "Tested by"() -> (w3491:string)
                n2718 = local read "String 33"() -> (w3492:string)
                n2719 = Concatenate Strings("," ("string"), "                                                                             " ("string")) -> (w3480:string)
                n2720 = Concatenate Strings(w3482, w3478, w3485, w3478, w3488, w3517, w3478, w3480, w3492, w3491) -> (→"export":string)
                n2721 = String To Path(string=w3519) -> (path=w3526:path)
                n2722 = local read "export"() -> (w3521:string)
                n2723 = call <vilib>:"Write Characters To File.vi"("append to file? (new file:F)"=FALSE, "character string"=w3521, "file path (dialog if empty)"=w3526) -> ()  [unwired: 2 in, 1 out]
              }
            }
          }
          frame Enabled {
          }
        }
        n2724 = case shown="True" "OK Button 17" {
          frame False {
          }
          frame True {
            (unwired) 0  # existing file
            w3779 = "Choose a datalog file to open"  # prompt
            n2725 = local write "OK Button 17"(FALSE ("OK Button 17")) -> ()
            n2726 = local read "String"() -> (w3774:string)
            n2727 = String To Path(string=w3774) -> (path=w3775:path)
            n2728 = File Dialog(6:"*.duf" ("pattern"), 7:w3779, 11:w3775) -> (0:w3766:errorcluster, 3:w3785:path)  [unwired: 4 in, 2 out]
            n2729 = Unbundle(w3766) -> ()  [unwired: 3 out]
            n2730 = Open/Create/Replace File "Open File"(file path (use dialog)=w3785) -> (refnum out=w3777:refnum<file>)  [unwired: 5 in, 2 out]
            n2731 = Strip Path(path=w3785) -> (name=w3783:string)  [unwired: 1 out]
